vi "Create Output File Name.vi"(8 "error in (no error)":errorcluster, 9 "Slot 2 Module Selection":T1, 10 "Slot 1 Module Selection":T1, 11 "Output Directory":path) -> (0 "error out":errorcluster, 3 "output file name":path)   [LabVIEW 2017]
uses:
  Slot Module Selection.ctl
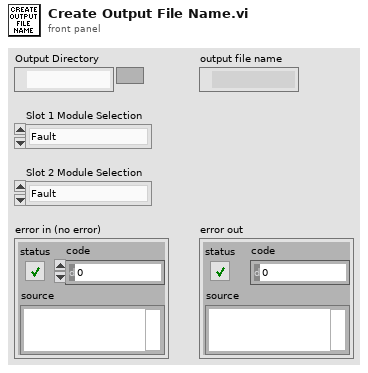
[diagram p1: front panel]
types:
  T1 = typedef "Slot Module Selection.ctl" = enum16{"Fault", "Instrument", "Empty"}
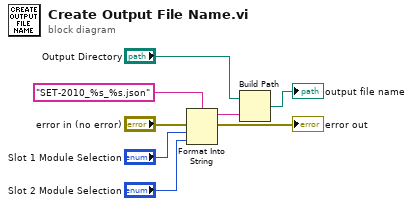
[diagram p0: block diagram]
diagram:
  n1 = Format Into String(format string="SET-2010_%s_%s.json", error in="error in (no error)", "Slot 1 Module Selection", "Slot 2 Module Selection") -> (resulting string=w5:string, error out=→"error out":errorcluster)  [unwired: 1 in]
  n2 = Build Path(base path="Output Directory", name or relative path=w5) -> (appended path=→"output file name":path)
